vi "svfa_Check Data Valid [Zoom] (1 Ch).vi"(0 "signal [V]":waveform(dbl), 1 "restart averaging (F)":bool, 9 "averaging parameters":T2={"averaging mode"=enum."No averaging", "weighting mode"=enum."Linear", "number of averages"=10, "linear mode"=enum."Auto restart"}, 11 "error in (no error)":errorcluster, 12 "zoom settings":T3={"frequency range"={"start frequency"=1000.0, "stop frequency"=2000.0}, "window"=1, "number of lines"=400, "% overlap"=0.0} {"% overlap" min=0.0 format="%.2f"; "number of lines" min=2; "window" items=["None ", "Hanning", "Hamming", "Blackman-Harris", "Exact Blackman", "Blackman", "Flat Top", "4 Term B-Harris ", "7 Term B-Harris", "Low Sidelobe"]; "frequency range"."stop frequency" min=0.0 format="%.2f"; "frequency range"."start frequency" min=0.0 format="%.2f"}) -> (2 "reset processing":bool, 3 "restart averaging":bool, 4 "dup signal [V]":waveform(dbl), 6 "iterations":i32, 8 "maximum block size":i32, 10 "dup averaging parameters":T2={"averaging mode"=enum."No averaging", "weighting mode"=enum."Linear", "number of averages"=10, "linear mode"=enum."Auto restart"}, 14 "zoom FFT settings":T1={"zoom settings"={"center frequency"=-inf, "zoom"=1, "trim"=1.0}, "FFT settings"={"window"=enum."Hanning", "window size"=-1, "FFT size"=1024, "%overlap"=0.0}} {"FFT settings"."%overlap" min=0.0 max=100.0 format="%.2f"; "zoom settings"."trim" min=1.0 format="%.2f"; "zoom settings"."center frequency" format="%.2f"; "zoom settings"."zoom" min=1}, 15 "error out":errorcluster)   [LabVIEW 2017]
uses:
  <vilib>/addons/_NISVFA/_Shared subVIs/Common/svc_Check for Waveform Parameter Continuity (no state).vi
  <vilib>/addons/_NISVFA/_Shared subVIs/Common/svc_Get SV Channel Info.vi
  <vilib>/addons/_NISVFA/_Shared subVIs/Common/svc_Engineering Units to Unit Label.vi
  <vilib>/addons/_NISVFA/_Shared subVIs/Common/svc_Unit Label to Engineering Units.vi
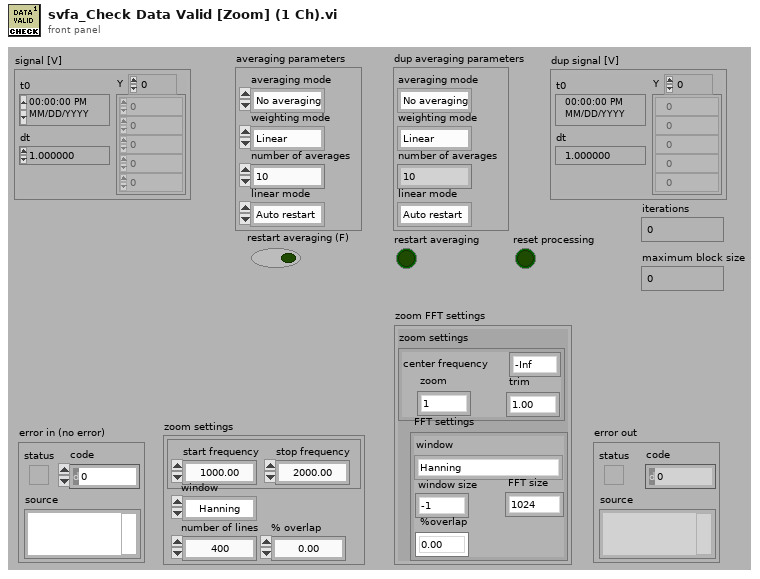
[diagram p1: front panel]
types:
  T1 = cluster{"zoom settings":cluster{"center frequency":dbl, "zoom":i32, "trim":dbl}, "FFT settings":cluster{"window":enum16{"None ", "Hanning", "Hamming", "Blackman-Harris", "Exact Blackman", "Blackman", "Flat Top", "4 Term B-Harris ", "7 Term B-Harris", "Low Sidelobe"}, "window size":i32, "FFT size":i32, "%overlap":dbl}}
  T2 = cluster{"averaging mode":enum16{"No averaging", "Vector averaging", "RMS averaging", "Peak hold"}, "weighting mode":enum16{"Linear", "Exponential"}, "number of averages":u32, "linear mode":enum16{"One shot", "Auto restart"}}
  T3 = cluster{"frequency range":cluster{"start frequency":dbl, "stop frequency":dbl}, "window":u16, "number of lines":i32, "% overlap":dbl}
  T4 = cluster{"dt":bool, "t0 continuity":bool, "array length":bool, "channel info":bool, "name":bool}
  T5 = typedef "NI_AALPro.lvlib/windowTd.ctl" = u32
  T6 = enum16{"No averaging", "Vector averaging", "RMS averaging", "Peak hold"}
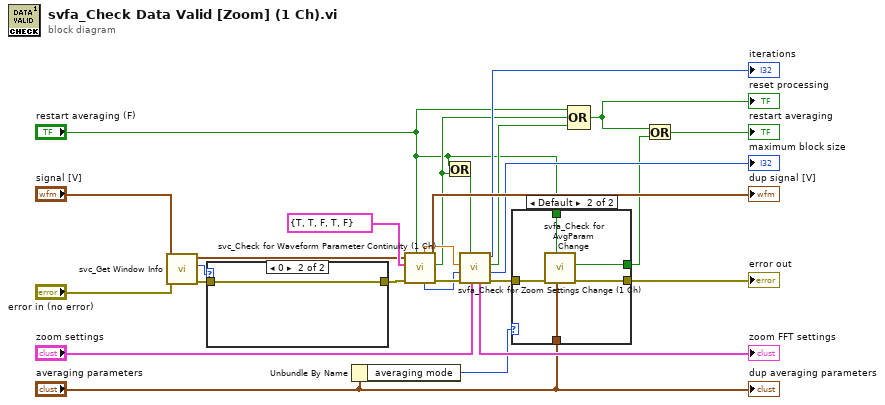
[diagram p0: block diagram]
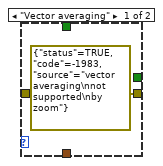
[diagram p2: hidden frame]
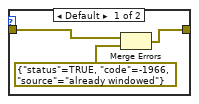
[diagram p3: hidden frame]
diagram:
  n1 = call <vilib>:"svc_Get Window Info.vi"("error in (no error)"="error in (no error)", "scaled signal [EU]"="signal [V]") -> ("error out"=w9:errorcluster, "window"=w10:T5, "dup scaled signal [EU]"=w11:waveform(dbl))  [unwired: 5 in, 2 out]
  n2 = case shown="0" w10 {
    tunnel: w9 -> [w28 w30]
    tunnel: [w29 w30] -> w8
    frame Default {
      n3 = Merge Errors(w28, errorcluster {"status"=TRUE, "code"=-1966, "source"="already windowed"} ("error in 2 (no error)")) -> (w29:errorcluster)
    }
    frame 0 {
    }
  }
  n4 = Unbundle By Name("averaging parameters") -> ("averaging mode"=w1:T6)
  n5 = call <vilib>:"svc_Check for Waveform Parameter Continuity (1 Ch).vi"("restart averaging (F)"="restart averaging (F)", "error in (no error)"=w8, "checks for channel parameter change"=T4 {"dt"=TRUE, "t0 continuity"=TRUE, "array length"=FALSE, "channel info"=TRUE, "name"=FALSE}, "scaled signal [EU]"=w11) -> ("error out"=w17:errorcluster, "waveform parameter changed"=w7:bool, "dup scaled signal [EU]"=→"dup signal [V]":waveform(dbl), "array length"=w12:i32, "dt"=w13:dbl)  [unwired: 2 in, 1 out]
  n6 = Or(x="restart averaging (F)", y=w7) -> (x .or. y?=w6:bool)
  n7 = call <vilib>:"svfa_Check for Zoom Settings Change (1 Ch).vi"("zoom settings"="zoom settings", "restart averaging (F)"=w6, "error in (no error)"=w17, "array length"=w12, "dt"=w13) -> ("error out"=w16:errorcluster, "maximum block size"=→"maximum block size":i32, "zoom settings changed"=w15:bool, "iterations"=→"iterations":i32, "zoom FFT settings"=→"zoom FFT settings":T1)  [unwired: 2 in]
  n8 = case shown="Default" w1 {
    tunnel: w16 -> [_ w36]
    tunnel: [_ w35] -> w5
    tunnel: "restart averaging (F)" -> [_ w34]
    tunnel: [errorcluster {"status"=TRUE, "code"=-1983, "source"="vector averaging\nnot supported\nby zoom"} ("error IO") w33] -> w3
    tunnel: "averaging parameters" -> [_ w32]
    frame "Vector averaging" {
    }
    frame Default {
      n9 = call <vilib>:"svfa_Check for AvgParam Change.vi"("averaging parameters"=w32, "restart averaging (F)"=w34, "error in (no error)"=w36) -> ("error out"=w33:errorcluster, "parameter has changed"=w35:bool)  [unwired: 7 in]
    }
  }
  "error out" <- w3
  n10 = Compound Arithmetic op=OR("restart averaging (F)", w7, w15) -> (w18:bool)
  "reset processing" <- w18
  n11 = Or(x=w18, y=w5) -> (x .or. y?=→"restart averaging":bool)
  "dup averaging parameters" <- "averaging parameters"
